vi "SetBusData.vi"(8 "Error In":errorcluster[](array[cluster]), 9 "XmlData":string, 10 "arg":string, 11 "Bus in":refnum<class "Bus.lvclass">) -> (0 "Error Out":errorcluster[](array[cluster]), 3 "Bus out":refnum<class "Bus.lvclass">)   [LabVIEW 2014, in "Bus_class.lvlib" / "Bus.lvclass"]
uses:
  Bus.lvclass
  Bus.lvclass/Bus.ctl
  Modules/EventModule/PublicAPI/Arguments/Requests/dblEvtParams.ctl
  Modules/EventPlugins/EventPluginBaseClass/TypeDefs/clEvtConfig.ctl
  Modules/PmuImpairPlugins/PmuImpairPluginBase_class/TypeDefs/clImpairConfig.ctl
  Modules/EventPlugins/EventPluginBaseClass/TypeDefs/clEvtReportArray.ctl
  Modules/EventPlugins/EventPluginBaseClass/TypeDefs/clEvtReport.ctl
  Modules/FlagImpairPlugins/FlagImpairPluginBase_class/TypeDefs/clFlagImpairConfig.ctl
  <vilib>/Utility/error.llb/Error Cluster From Error Code.vi
  <vilib>/ErrorRing/Error Ring.xnode
  TestAutomation/LTA/LTA.lvlib
  <userlib>/NIST/NISTErrorLib/NISTErrorLib.lvlib
  Modules/EventModule/EventModule.lvlib
  Modules/EventPlugins/EventPluginBaseClass/EventPluginBaseClass.lvclass
  Modules/PmuImpairPlugins/PmuImpairPluginBase_class/PmuImpairPluginBase.lvclass
  Modules/PmuImpairModule/PmuImpairModule.lvlib
  Modules/NetworkImpairmentModule/NetworkImpairmentModule.lvlib
  Modules/FlagImpairModule/FlagImpairModule.lvlib
  Modules/FlagImpairPlugins/FlagImpairPluginBase_class/FlagImpairPluginBase.lvclass
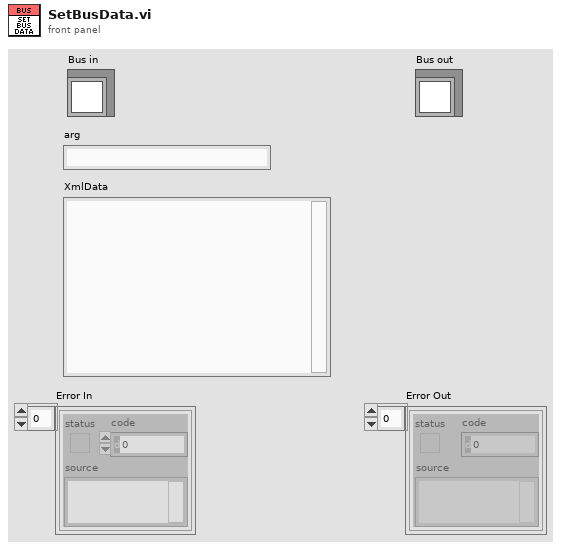
[diagram p1: front panel]
types:
  T1 = typedef "EventPlugins.lvlib/EventPluginBaseClass.lvclass/clEvtConfig.ctl" = cluster{"T0(UTC)":dbl, "F0":dbl, "Fs":i32, "FSamp":u32, "bPosSeq":bool}
  T2 = typedef "EventModule.lvlib/dblEvtParams.ctl" = dbl[][]
  T3 = typedef "PmuImpairPlugins.lvlib/PmuImpairPluginBase.lvclass/clImpairConfig.ctl" = cluster{"FilterType":string, "bPosSeq":bool}
  T4 = typedef "EventPlugins.lvlib/EventPluginBaseClass.lvclass/clEvtReportArray.ctl" = T5[]
  T5 = typedef "EventPlugins.lvlib/EventPluginBaseClass.lvclass/clEvtReport.ctl" = cluster{"Timestamp":dbl, "Synx":cdb[], "Freq":dbl, "ROCOF":dbl, "ID":i16}
  T6 = typedef "FlagImpairPlugins.lvlib/FlagImpairPluginBase.lvclass/clFlagImpairConfig.ctl" = cluster{"FlagImpairmentType":u16}
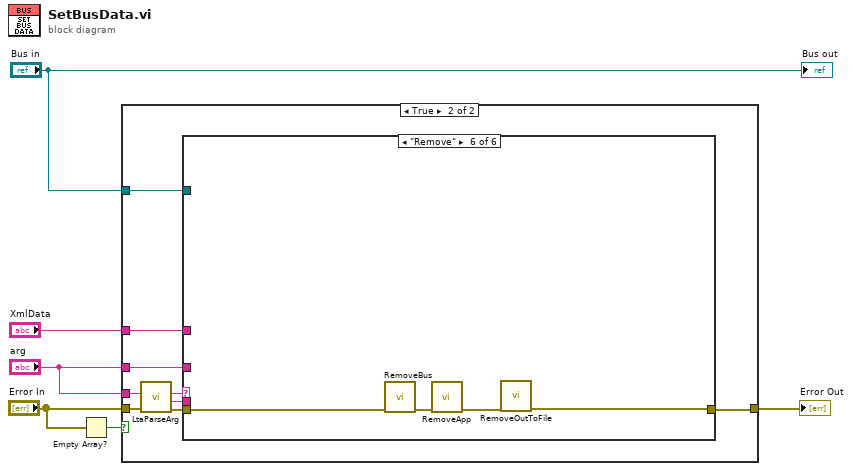
[diagram p0: block diagram]
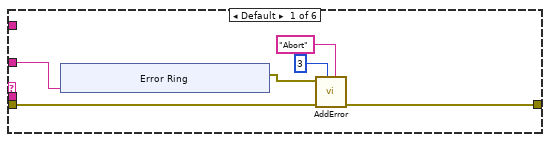
[diagram p3: hidden frame]
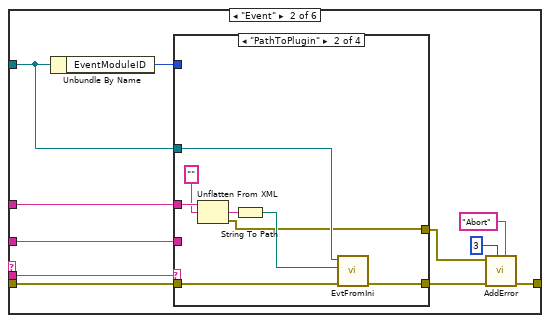
[diagram p4: hidden frame]
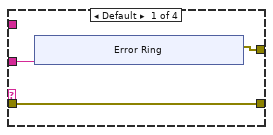
[diagram p5: hidden frame]
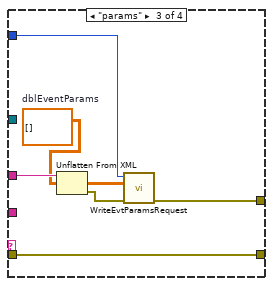
[diagram p6: hidden frame]
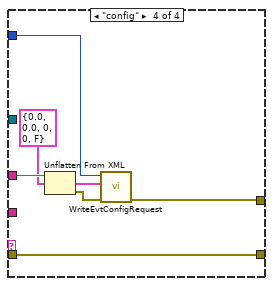
[diagram p7: hidden frame]
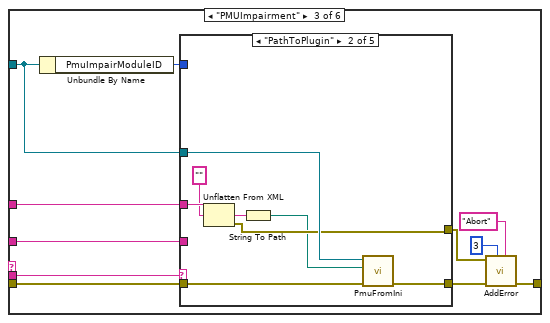
[diagram p8: hidden frame]
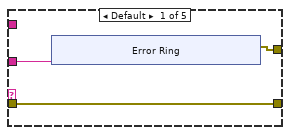
[diagram p9: hidden frame]
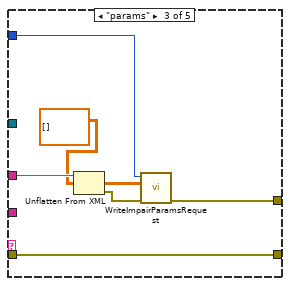
[diagram p10: hidden frame]
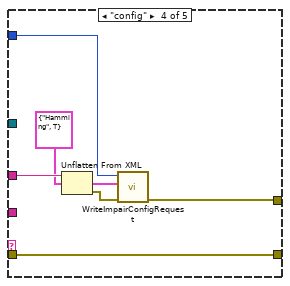
[diagram p11: hidden frame]
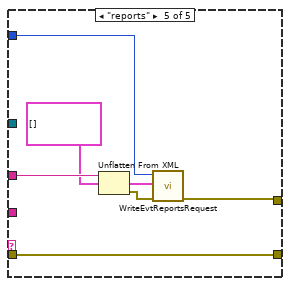
[diagram p12: hidden frame]
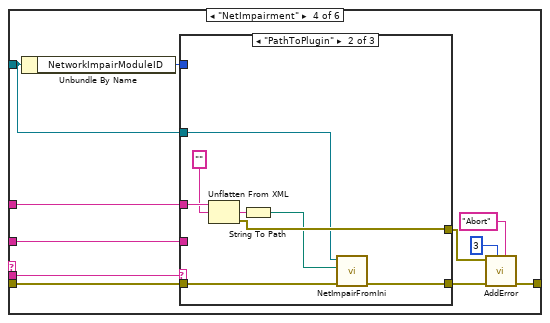
[diagram p13: hidden frame]
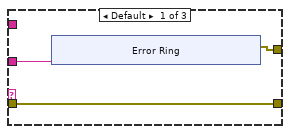
[diagram p14: hidden frame]
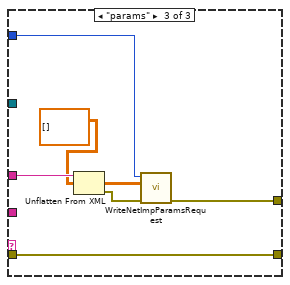
[diagram p15: hidden frame]
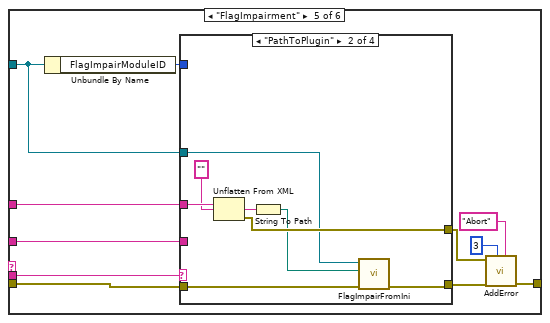
[diagram p16: hidden frame]
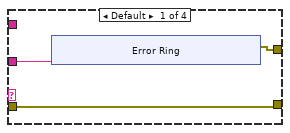
[diagram p17: hidden frame]
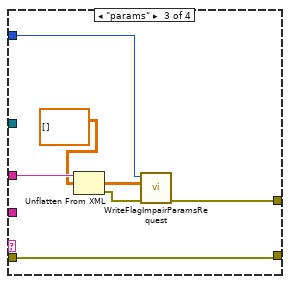
[diagram p18: hidden frame]
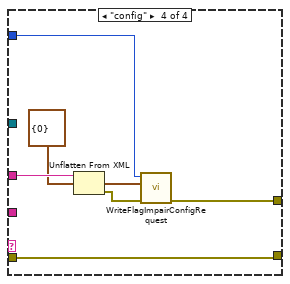
[diagram p19: hidden frame]
diagram:
  n1 = Empty Array?(array="Error In") -> (empty?=w6:bool)
  n2 = case shown="True" w6 {
    tunnel: "Error In" -> [w7 w16]
    tunnel: [w7 w11] -> w4
    tunnel: "arg" -> [_ w15]
    tunnel: "Bus in" -> [_ w10]
    tunnel: "arg" -> [_ w9]
    tunnel: "XmlData" -> [_ w8]
    frame False {
    }
    frame True {
      n3 = call "LtaParseArg.vi"("Error In"=w16, "Arg In"=w15) -> ("Error Out"=w13:errorcluster[], "ArgRemaining"=w12:string, "Arg 1"=w14:string)  [unwired: 6 in, 1 out]
      n4 = case shown="\"Remove\"" w14 {
        tunnel: w13 -> [w20 w32 w75 w125 w160 w203]
        tunnel: w12 -> [_ w40 w83 w133 w169 _]
        tunnel: [w18 w34 w77 w127 w163 w202] -> w11
        tunnel: w10 -> [_ w30 w73 w123 w161 _]
        tunnel: w9 -> [w17 w39 w82 w132 w168 _]
        tunnel: w8 -> [_ w37 w80 w130 w166 _]
        frame Default {
          n5 = xnode "Error Ring"("parameter 0"=w17) -> ("error out"=w19:errorcluster)
          n6 = call <userlib>:"AddError.vi"("Severity"="Abort", "Priority"=u8 3, "ErrorArray"=w20, "error in (no error)"=w19) -> ("ErrorArray"=w18:errorcluster[])  [unwired: 6 in, 1 out]
        }
        frame "Event" {
          n7 = Unbundle By Name(w30) -> ("EventModuleID"=w38:i32)
          n8 = case shown="\"PathToPlugin\"" w40 {
            tunnel: w39 -> [w43 _ _ _]
            tunnel: w38 -> [_ _ w61 w68]
            tunnel: w37 -> [_ w58 w65 w72]
            tunnel: [w42 w51 w60 w67] -> w33
            tunnel: w32 -> [w41 w55 w59 w66]
            tunnel: [w41 w54 w59 w66] -> w31
            tunnel: w30 -> [_ w53 _ _]
            frame Default {
              n9 = xnode "Error Ring"("parameter 0"=w43) -> ("error out"=w42:errorcluster)
            }
            frame "PathToPlugin" {
              n10 = Unflatten From XML(xml string=w58, type="") -> (value=w56:string, error out=w51:errorcluster)  [unwired: 1 in]
              n11 = String To Path(string=w56) -> (path=w52:path)
              n12 = call "EvtFromIni.vi"("ErrorArray In"=w55, "PathToIni"=w52, "Bus in"=w53) -> ("ErrorArray Out"=w54:errorcluster[])  [unwired: 7 in, 1 out]
            }
            frame "params" {
              w64 = T2 []  # dblEventParams
              n13 = Unflatten From XML(xml string=w65, type=w64) -> (value=w63:T2, error out=w62:errorcluster)  [unwired: 1 in]
              n14 = call "WriteEvtParamsRequest.vi"("error in (no error)"=w62, "EvtParams"=w63, "ModuleID"=w61) -> ("error out"=w60:errorcluster)  [unwired: 8 in]
            }
            frame "config" {
              n15 = Unflatten From XML(xml string=w72, type=T1 {"T0(UTC)"=0.0, "F0"=0.0, "Fs"=0, "FSamp"=0, "bPosSeq"=FALSE} ("clEvtConfig")) -> (value=w70:T1, error out=w69:errorcluster)  [unwired: 1 in]
              n16 = call "WriteEvtConfigRequest.vi"("error in (no error)"=w69, "clEvtConfig"=w70, "ModuleID"=w68) -> ("error out"=w67:errorcluster)  [unwired: 8 in]
            }
          }
          n17 = call <userlib>:"AddError.vi"("Severity"="Abort", "Priority"=u8 3, "ErrorArray"=w31, "error in (no error)"=w33) -> ("ErrorArray"=w34:errorcluster[])  [unwired: 6 in, 1 out]
        }
        frame "PMUImpairment" {
          n18 = Unbundle By Name(w73) -> ("PmuImpairModuleID"=w81:i32)
          n19 = case shown="\"PathToPlugin\"" w83 {
            tunnel: w82 -> [w86 _ _ _ _]
            tunnel: w81 -> [_ _ w104 w112 w119]
            tunnel: w80 -> [_ w101 w108 w115 w122]
            tunnel: [w85 w95 w103 w111 w117] -> w76
            tunnel: w75 -> [w84 w98 w102 w109 w116]
            tunnel: [w84 w97 w102 w109 w116] -> w74
            tunnel: w73 -> [_ w96 _ _ _]
            frame Default {
              n20 = xnode "Error Ring"("parameter 0"=w86) -> ("error out"=w85:errorcluster)
            }
            frame "PathToPlugin" {
              n21 = Unflatten From XML(xml string=w101, type="") -> (value=w99:string, error out=w95:errorcluster)  [unwired: 1 in]
              n22 = String To Path(string=w99) -> (path=w94:path)
              n23 = call "PmuFromIni.vi"("ErrorArray In"=w98, "PathToIni"=w94, "Bus in"=w96) -> ("ErrorArray Out"=w97:errorcluster[])  [unwired: 7 in, 1 out]
            }
            frame "params" {
              n24 = Unflatten From XML(xml string=w108, type=T2 [] ("dblEventParams")) -> (value=w106:T2, error out=w105:errorcluster)  [unwired: 1 in]
              n25 = call "WriteImpairParamsRequest.vi"("error in (no error)"=w105, "dblImpairParams"=w106, "ModuleID"=w104) -> ("error out"=w103:errorcluster)  [unwired: 8 in]
            }
            frame "config" {
              n26 = Unflatten From XML(xml string=w115, type=T3 {"FilterType"="Hamming", "bPosSeq"=TRUE} ("clImpairConfig")) -> (value=w110:T3, error out=w113:errorcluster)  [unwired: 1 in]
              n27 = call "WriteImpairConfigRequest.vi"("error in (no error)"=w113, "clImpairConfig"=w110, "ModuleID"=w112) -> ("error out"=w111:errorcluster)  [unwired: 8 in]
            }
            frame "reports" {
              n28 = Unflatten From XML(xml string=w122, type=T4 [] ("clEvtReportArray")) -> (value=w120:T4, error out=w118:errorcluster)  [unwired: 1 in]
              n29 = call "WriteEvtReportsRequest.vi"("error in (no error)"=w118, "EvtReportArray"=w120, "ModuleID"=w119) -> ("error out"=w117:errorcluster)  [unwired: 8 in]
            }
          }
          n30 = call <userlib>:"AddError.vi"("Severity"="Abort", "Priority"=u8 3, "ErrorArray"=w74, "error in (no error)"=w76) -> ("ErrorArray"=w77:errorcluster[])  [unwired: 6 in, 1 out]
        }
        frame "NetImpairment" {
          n31 = Unbundle By Name(w123) -> ("NetworkImpairModuleID"=w131:i32)
          n32 = case shown="\"PathToPlugin\"" w133 {
            tunnel: w132 -> [w136 _ _]
            tunnel: w131 -> [_ _ w154]
            tunnel: w130 -> [_ w151 w158]
            tunnel: [w135 w148 w153] -> w126
            tunnel: w125 -> [w134 w147 w152]
            tunnel: [w134 w146 w152] -> w124
            tunnel: w123 -> [_ w145 _]
            frame Default {
              n33 = xnode "Error Ring"("parameter 0"=w136) -> ("error out"=w135:errorcluster)
            }
            frame "PathToPlugin" {
              n34 = Unflatten From XML(xml string=w151, type="") -> (value=w149:string, error out=w148:errorcluster)  [unwired: 1 in]
              n35 = String To Path(string=w149) -> (path=w144:path)
              n36 = call "NetImpairFromIni.vi"("ErrorArray In"=w147, "PathToIni"=w144, "Bus in"=w145) -> ("ErrorArray Out"=w146:errorcluster[])  [unwired: 7 in, 1 out]
            }
            frame "params" {
              n37 = Unflatten From XML(xml string=w158, type=T2 [] ("dblEventParams")) -> (value=w156:T2, error out=w155:errorcluster)  [unwired: 1 in]
              n38 = call "WriteNetImpParamsRequest.vi"("error in (no error)"=w155, "dblNetImpParams"=w156, "ModuleID"=w154) -> ("error out"=w153:errorcluster)  [unwired: 8 in]
            }
          }
          n39 = call <userlib>:"AddError.vi"("Severity"="Abort", "Priority"=u8 3, "ErrorArray"=w124, "error in (no error)"=w126) -> ("ErrorArray"=w127:errorcluster[])  [unwired: 6 in, 1 out]
        }
        frame "FlagImpairment" {
          n40 = Unbundle By Name(w161) -> ("FlagImpairModuleID"=w167:i32)
          n41 = case shown="\"PathToPlugin\"" w169 {
            tunnel: w168 -> [w172 _ _ _]
            tunnel: w167 -> [_ _ w190 w199]
            tunnel: w166 -> [_ w187 w194 w201]
            tunnel: [w171 w182 w189 w198] -> w162
            tunnel: w161 -> [_ w180 _ _]
            tunnel: [w170 w183 w188 w195] -> w159
            tunnel: w160 -> [w170 w184 w188 w195]
            frame Default {
              n42 = xnode "Error Ring"("parameter 0"=w172) -> ("error out"=w171:errorcluster)
            }
            frame "PathToPlugin" {
              n43 = Unflatten From XML(xml string=w187, type="") -> (value=w185:string, error out=w182:errorcluster)  [unwired: 1 in]
              n44 = String To Path(string=w185) -> (path=w181:path)
              n45 = call "FlagImpairFromIni.vi"("ErrorArray In"=w184, "PathToIni"=w181, "Bus in"=w180) -> ("ErrorArray Out"=w183:errorcluster[])  [unwired: 7 in, 1 out]
            }
            frame "params" {
              n46 = Unflatten From XML(xml string=w194, type=T2 [] ("dblEventParams")) -> (value=w192:T2, error out=w191:errorcluster)  [unwired: 1 in]
              n47 = call "WriteFlagImpairParamsRequest.vi"("error in (no error)"=w191, "dblFlagImpairParams"=w192, "ModuleID"=w190) -> ("error out"=w189:errorcluster)  [unwired: 8 in]
            }
            frame "config" {
              n48 = Unflatten From XML(xml string=w201, type=T6 {"FlagImpairmentType"=0} ("clFlagImpairConfig")) -> (value=w196:T6, error out=w200:errorcluster)  [unwired: 1 in]
              n49 = call "WriteFlagImpairConfigRequest.vi"("error in (no error)"=w200, "clFlagImpairConfig"=w196, "ModuleID"=w199) -> ("error out"=w198:errorcluster)  [unwired: 8 in]
            }
          }
          n50 = call <userlib>:"AddError.vi"("Severity"="Abort", "Priority"=u8 3, "ErrorArray"=w159, "error in (no error)"=w162) -> ("ErrorArray"=w163:errorcluster[])  [unwired: 6 in, 1 out]
        }
        frame "Remove" {
          n51 = call "RemoveBus.vi"("ErrorArray In"=w203) -> ("ErrorArray Out"=w205:errorcluster[])  [unwired: 10 in]
          n52 = call "RemoveApp.vi"("ErrorArray In"=w205) -> ("ErrorArray Out"=w204:errorcluster[])  [unwired: 10 in]
          n53 = call "RemoveOutToFile.vi"("ErrorArray In"=w204) -> ("ErrorArray Out"=w202:errorcluster[])  [unwired: 10 in]
        }
      }
    }
  }
  "Error Out" <- w4
  "Bus out" <- "Bus in"
